vi "GUI AC Source setup.vi"(10 "AC sync source":T2, 11 "AC Source":T2) -> (2 "AC sync source out":T2, 3 "AC Source out":T2)   [LabVIEW 2020]
doc: "GUI to set up the AC source and check connection."
uses:
  General AC source/Type definitions/AC Source.ctl
  General AC source/Type definitions/AC Source type.ctl
  <vilib>/Utility/error.llb/DialogType.ctl
  <vilib>/Utility/error.llb/Error Cluster From Error Code.vi
  <vilib>/ErrorRing/Error Ring.xnode
  external libraries/varilib/varilib.lvlib
panel:
  in  "AC sync Fluke 57XX ignore errors":bool
  in  "Fluke 57XX ignore errors":bool
  out "sync not tested label":string="This device is not yet fully tested!"
  in  "AC sync VISA":refnum<visa-resource-name> caption="VISA"
  in  "AC sync Fluke 57XX wideband output":bool caption="Fluke 57XX wideband output"
  in  "AC sync ref. clock (Hz)":dbl caption="Reference clock (Hz)\nIf set to zero, ref. clock\nis not used." format="%#_6p"
  in  "AC sync type":T1 caption="AC synchronization type"
  in  "Synchronization by AC signal":bool
  in  "Fluke 57XX wideband output":bool
  out "not tested label":string="This device is not yet fully tested!"
  in  "Ref. clock (Hz)":dbl caption="Reference clock (Hz)\nIf set to zero, ref. clock\nis not used." format="%#_6p"
  in  "AC source type":T1
  in  "VISA":refnum<visa-resource-name>
  out "gui_elements":refnum<vi>[](array[refnum])
  out "Status":string
  in  "save_and_quit":bool
  in  "test":bool
  in  "cancel":bool
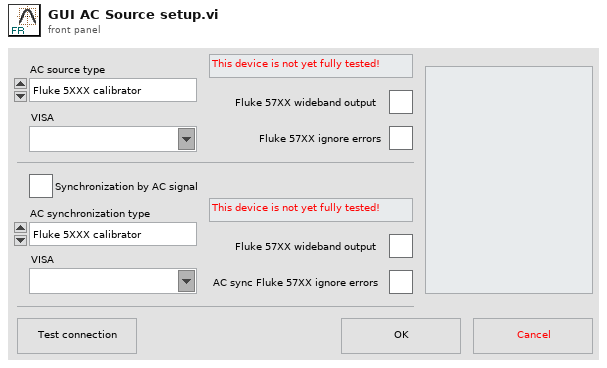
[diagram p1: front panel]
types:
  T1 = typedef "AC Source type.ctl" = enum16{"Fluke 5XXX calibrator", "Tektronix AFG3000 series", "dummy", "Agilent 331xxA to 332xxA", "Agilent 335xxA to 336xxA"}
  T2 = typedef "AC Source.ctl" = cluster{"AC Source type":T1, "VISA":refnum<visa-resource-name>, "Ref. clock (Hz)":dbl, "status ref":refnum<vi>, "Fluke 57XX wideband output":bool, "Fluke 57XX ignore errors":bool, "Synchronization by AC signal":bool}
  T3 = typedef "DialogType.ctl" = u16
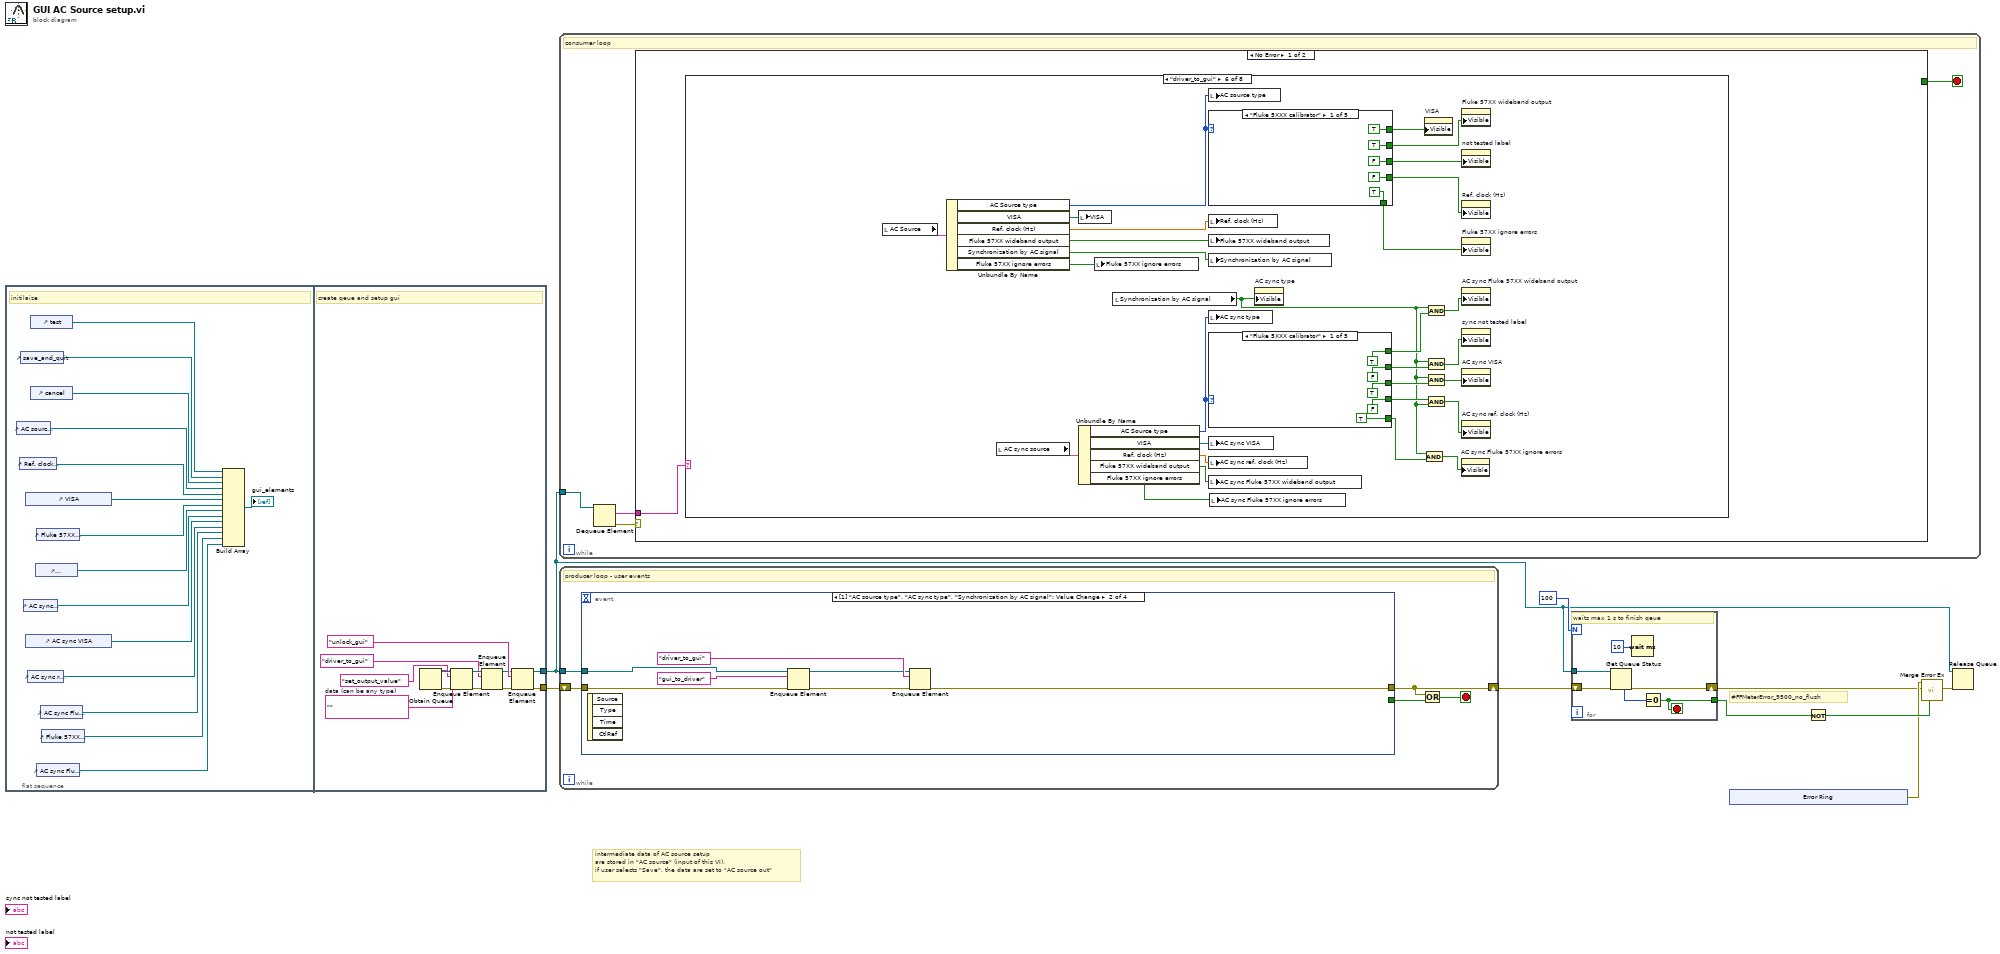
[diagram p0: block diagram]
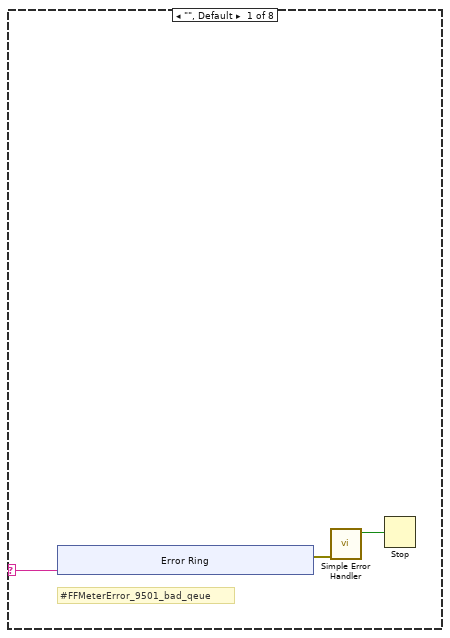
[diagram p2: hidden frame]
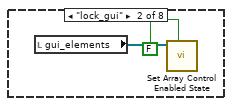
[diagram p3: hidden frame]
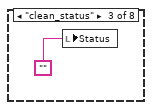
[diagram p4: hidden frame]
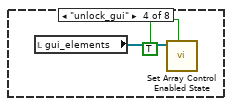
[diagram p5: hidden frame]
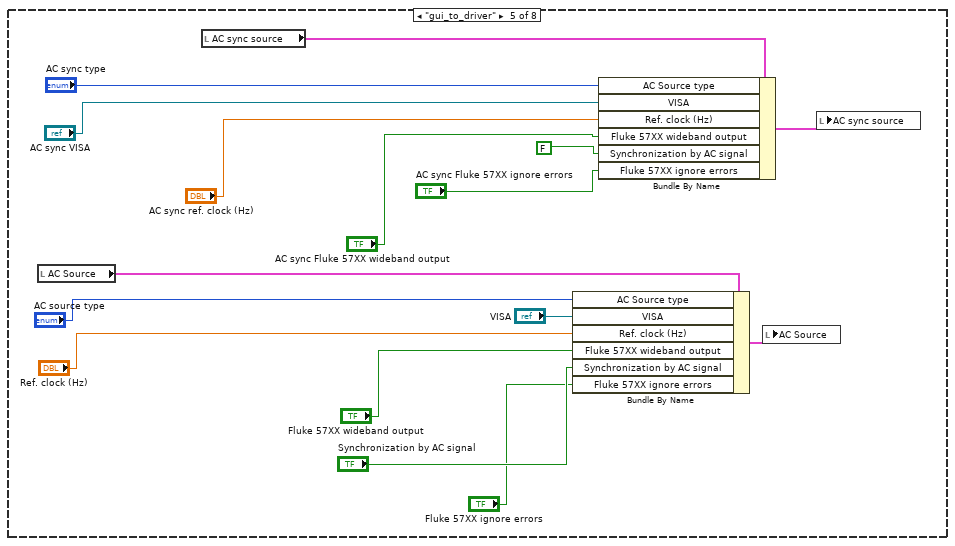
[diagram p6: hidden frame]
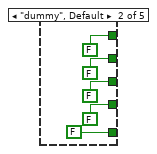
[diagram p7: hidden frame]
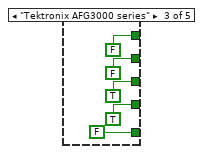
[diagram p8: hidden frame]
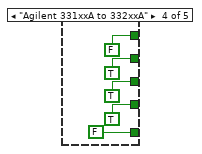
[diagram p9: hidden frame]
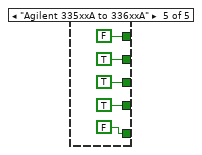
[diagram p10: hidden frame]
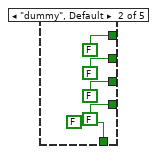
[diagram p11: hidden frame]
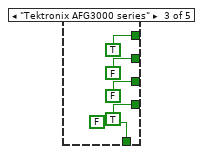
[diagram p12: hidden frame]
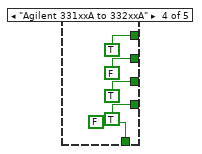
[diagram p13: hidden frame]
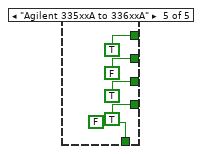
[diagram p14: hidden frame]
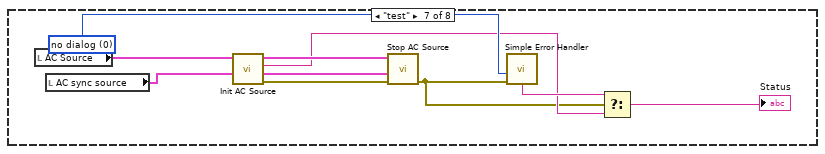
[diagram p15: hidden frame]
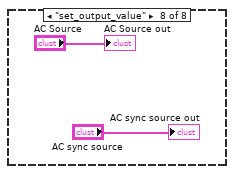
[diagram p16: hidden frame]
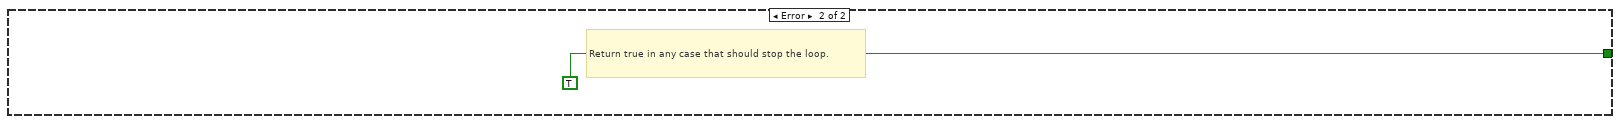
[diagram p17: hidden frame]
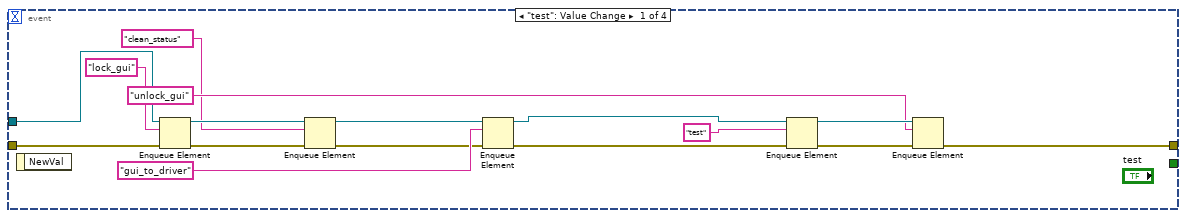
[diagram p18: hidden frame]
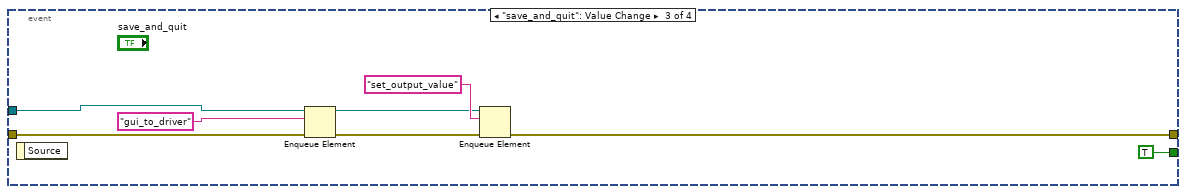
[diagram p19: hidden frame]
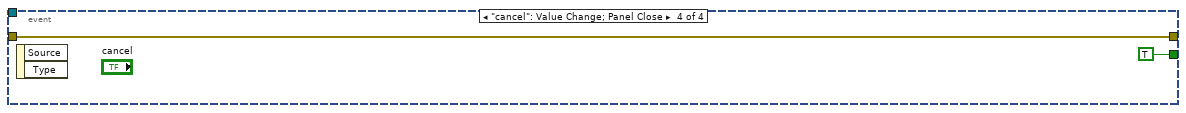
[diagram p20: hidden frame]
diagram:
  # "#FFMeterError_9500_no_flush"
  # "intermediate data of AC source setup\nare stored in \"AC source\" (input of this VI),\nif user selects \"Save\", the data are set to \"AC source out\""
  n1 = flat-sequence {
    tunnel: [w29] -> w2
    tunnel: [w27] -> w1
    frame #0 {
      # "initilaize"
      n2 = control-ref of="AC source type"() -> (w19:refnum<vi>)
      n3 = control-ref of="Ref. clock (Hz)"() -> (w18:refnum<vi>)
      n4 = control-ref of="save_and_quit"() -> (w23:refnum<vi>)
      n5 = control-ref of="AC sync type"() -> (w15:refnum<vi>)
      n6 = control-ref of="VISA"() -> (w20:refnum<vi>)
      n7 = control-ref of="AC sync VISA"() -> (w14:refnum<vi>)
      n8 = control-ref of="AC sync ref. clock (Hz)"() -> (w13:refnum<vi>)
      n9 = control-ref of="test"() -> (w24:refnum<vi>)
      n10 = control-ref of="cancel"() -> (w22:refnum<vi>)
      n11 = control-ref of="Synchronization by AC signal"() -> (w16:refnum<vi>)
      n12 = control-ref of="Fluke 57XX wideband output"() -> (w17:refnum<vi>)
      n13 = control-ref of="AC sync Fluke 57XX ignore errors"() -> (w10:refnum<vi>)
      n14 = control-ref of="AC sync Fluke 57XX wideband output"() -> (w12:refnum<vi>)
      n15 = control-ref of="Fluke 57XX ignore errors"() -> (w11:refnum<vi>)
      n16 = Build Array(w24, w23, w22, w19, w18, w20, w17, w16, w15, w14, w13, w12, w11, w10) -> (→"gui_elements":refnum<vi>[])
    }
    frame #1 {
      w28 = ""  # data (can be any type)
      # "create qeue and setup gui"
      n17 = Obtain Queue(element data type=w28) -> (queue out=w33:refnum<queue>, error out=w35:errorcluster)  [unwired: 4 in, 1 out]
      n18 = Enqueue Element(queue=w33, element="set_output_value", error in (no error)=w35) -> (queue out=w34:refnum<queue>, error out=w36:errorcluster)  [unwired: 1 in, 1 out]
      n19 = Enqueue Element(queue=w34, element="driver_to_gui", error in (no error)=w36) -> (queue out=w25:refnum<queue>, error out=w26:errorcluster)  [unwired: 1 in, 1 out]
      n20 = Enqueue Element(queue=w25, element="unlock_gui", error in (no error)=w26) -> (queue out=w29:refnum<queue>, error out=w27:errorcluster)  [unwired: 1 in, 1 out]
    }
  }
  n21 = while {
    tunnel: w2 -> [w40]
    stop <- w37 stop-if-true
    # "consumer loop"
    n22 = Dequeue Element(queue=w40) -> (element=w38:string, error out=w39:errorcluster)  [unwired: 2 in, 2 out]
    n23 = case shown="No Error" w39 {
      tunnel: w38 -> [w41 _]
      tunnel: [_ TRUE] -> w37
      frame No Error {
        n24 = case shown="\"driver_to_gui\"" w41 {
          selector: w41 -> [w42 _ _ _ _ _ _ _]
          frame "", Default {
            # "#FFMeterError_9501_bad_qeue"
            n25 = xnode "Error Ring"("parameter 0"=w42) -> ("error out"=w44:errorcluster)
            n26 = call <vilib>:"Simple Error Handler.vi"("error in (no error)"=w44) -> ("error?"=w43:bool)  [unwired: 4 in, 4 out]
            n27 = Stop(stop? (T)=w43) -> ()
          }
          frame "lock_gui" {
            n28 = local read "gui_elements"() -> (w53:refnum<vi>[])
            n29 = call "Set Array Control Enabled State.vi"("enabled (T)"=FALSE, "reference array in"=w53) -> ()  [unwired: 8 in, 2 out]
          }
          frame "clean_status" {
            n30 = local write "Status"("") -> ()
          }
          frame "unlock_gui" {
            n31 = local read "gui_elements"() -> (w56:refnum<vi>[])
            n32 = call "Set Array Control Enabled State.vi"("enabled (T)"=TRUE, "reference array in"=w56) -> ()  [unwired: 8 in, 2 out]
          }
          frame "gui_to_driver" {
            n33 = local read "AC Source"() -> (w71:T2)
            n34 = local read "AC sync source"() -> (w65:T2)
            n35 = Bundle By Name(cluster=w71, "AC Source type"="AC source type", "VISA"="VISA", "Ref. clock (Hz)"="Ref. clock (Hz)", "Fluke 57XX wideband output"="Fluke 57XX wideband output", "Synchronization by AC signal"="Synchronization by AC signal", "Fluke 57XX ignore errors"="Fluke 57XX ignore errors") -> (w72:T2)
            n36 = Bundle By Name(cluster=w65, "AC Source type"="AC sync type", "VISA"="AC sync VISA", "Ref. clock (Hz)"="AC sync ref. clock (Hz)", "Fluke 57XX wideband output"="AC sync Fluke 57XX wideband output", "Synchronization by AC signal"=FALSE, "Fluke 57XX ignore errors"="AC sync Fluke 57XX ignore errors") -> (w66:T2)
            n37 = local write "AC Source"(w72) -> ()
            n38 = local write "AC sync source"(w66) -> ()
          }
          frame "driver_to_gui" {
            n39 = local read "AC Source"() -> (w101:T2)
            n40 = Unbundle By Name(w101) -> ("AC Source type"=w100:T1, "VISA"=w97:refnum<visa-resource-name>, "Ref. clock (Hz)"=w99:dbl, "Fluke 57XX wideband output"=w94:bool, "Synchronization by AC signal"=w79:bool, "Fluke 57XX ignore errors"=w78:bool)
            n41 = local read "AC sync source"() -> (w92:T2)
            n42 = local write "VISA"(w97) -> ()
            n43 = Unbundle By Name(w92) -> ("AC Source type"=w88:T1, "VISA"=w91:refnum<visa-resource-name>, "Ref. clock (Hz)"=w90:dbl, "Fluke 57XX wideband output"=w89:bool, "Fluke 57XX ignore errors"=w77:bool)
            n44 = local write "Fluke 57XX ignore errors"(w78) -> ()
            n45 = local read "Synchronization by AC signal"() -> (w75:bool)
            n46 = local write "AC source type"(w100) -> ()
            n47 = case shown="\"Fluke 5XXX calibrator\"" w100 {
              tunnel: [FALSE ("x") FALSE ("x") TRUE ("x") TRUE ("x") TRUE ("x")] -> w96
              tunnel: [TRUE ("x") FALSE ("x") TRUE ("x") TRUE ("x") TRUE ("x")] -> w98
              tunnel: [FALSE ("x") FALSE ("x") FALSE ("x") TRUE ("x") TRUE ("x")] -> w95
              tunnel: [TRUE ("x") FALSE ("x") FALSE ("x") FALSE ("x") FALSE ("x")] -> w93
              tunnel: [TRUE ("x") FALSE ("x") FALSE ("x") FALSE ("x") FALSE ("x")] -> w76
              frame "Fluke 5XXX calibrator" {
              }
              frame "dummy", Default {
              }
              frame "Tektronix AFG3000 series" {
              }
              frame "Agilent 331xxA to 332xxA" {
              }
              frame "Agilent 335xxA to 336xxA" {
              }
            }
            n48 = local write "Ref. clock (Hz)"(w99) -> ()
            n49 = local write "Fluke 57XX wideband output"(w94) -> ()
            n50 = local write "Synchronization by AC signal"(w79) -> ()
            n51 = local write "AC sync type"(w88) -> ()
            n52 = case shown="\"Fluke 5XXX calibrator\"" w88 {
              tunnel: [FALSE ("x") FALSE ("x") TRUE ("x") TRUE ("x") TRUE ("x")] -> w83
              tunnel: [TRUE ("x") FALSE ("x") TRUE ("x") TRUE ("x") TRUE ("x")] -> w87
              tunnel: [FALSE ("x") FALSE ("x") FALSE ("x") TRUE ("x") TRUE ("x")] -> w85
              tunnel: [TRUE ("x") FALSE ("x") FALSE ("x") FALSE ("x") FALSE ("x")] -> w81
              tunnel: [TRUE ("x") FALSE ("x") FALSE ("x") FALSE ("x") FALSE ("x")] -> w74
              frame "Fluke 5XXX calibrator" {
              }
              frame "dummy", Default {
              }
              frame "Tektronix AFG3000 series" {
              }
              frame "Agilent 331xxA to 332xxA" {
              }
              frame "Agilent 335xxA to 336xxA" {
              }
            }
            n53 = local write "AC sync VISA"(w91) -> ()
            n54 = local write "AC sync ref. clock (Hz)"(w90) -> ()
            n55 = local write "AC sync Fluke 57XX wideband output"(w89) -> ()
            n56 = local write "AC sync Fluke 57XX ignore errors"(w77) -> ()
            n57 = property on="AC sync type" class="Enum (strict)"("Visible"=w75) -> ()  [unwired: 2 in, 2 out]
            n58 = And(x=w75, y=w74) -> (x .and. y?=w73:bool)
            n59 = property on="VISA" class="VISAName"("Visible"=w98) -> ()  [unwired: 2 in, 2 out]
            n60 = And(x=w75, y=w81) -> (x .and. y?=w80:bool)
            n61 = And(x=w75, y=w85) -> (x .and. y?=w84:bool)
            n62 = And(x=w75, y=w87) -> (x .and. y?=w86:bool)
            n63 = And(x=w83, y=w75) -> (x .and. y?=w82:bool)
            n64 = property on="AC sync Fluke 57XX ignore errors" class="Bool (strict)"("Visible"=w73) -> ()  [unwired: 2 in, 2 out]
            n65 = property on="Fluke 57XX wideband output" class="Bool (strict)"("Visible"=w93) -> ()  [unwired: 2 in, 2 out]
            n66 = property on="not tested label" class="Str"("Visible"=w95) -> ()  [unwired: 2 in, 2 out]
            n67 = property on="Ref. clock (Hz)" class="DigNum (strict)"("Visible"=w96) -> ()  [unwired: 2 in, 2 out]
            n68 = property on="Fluke 57XX ignore errors" class="Bool (strict)"("Visible"=w76) -> ()  [unwired: 2 in, 2 out]
            n69 = property on="AC sync Fluke 57XX wideband output" class="Bool (strict)"("Visible"=w80) -> ()  [unwired: 2 in, 2 out]
            n70 = property on="sync not tested label" class="Str"("Visible"=w84) -> ()  [unwired: 2 in, 2 out]
            n71 = property on="AC sync VISA" class="VISAName"("Visible"=w86) -> ()  [unwired: 2 in, 2 out]
            n72 = property on="AC sync ref. clock (Hz)" class="DigNum (strict)"("Visible"=w82) -> ()  [unwired: 2 in, 2 out]
          }
          frame "test" {
            w161 = T3 0 items=["no dialog", "OK message", "continue or stop message", "OK message + warnings", "continue/stop + warnings"] ("type of dialog (OK msg:1)")
            n73 = local read "AC Source"() -> (w158:T2)
            n74 = local read "AC sync source"() -> (w153:T2)
            n75 = call "Init AC Source.vi"("AC sync source"=w153, "AC source"=w158) -> ("error out"=w156:errorcluster, "AC sync source out"=w152:T2, "Init status"=w155:string, "AC source out"=w157:T2)  [unwired: 6 in]
            n76 = call "Stop AC Source.vi"("error in (no error)"=w156, "AC sync source"=w152, "AC source"=w157) -> ("error out"=w154:errorcluster)  [unwired: 6 in, 2 out]
            n77 = call <vilib>:"Simple Error Handler.vi"("type of dialog (OK msg:1)"=w161, "error in (no error)"=w154) -> ("message"=w160:string)  [unwired: 3 in, 4 out]
            n78 = Select(t=w160, s=w154, f=w155) -> (s? t:f=→"Status":string)
          }
          frame "set_output_value" {
            "AC Source out" <- "AC Source"
            "AC sync source out" <- "AC sync source"
          }
        }
      }
      frame Error {
        # "Return true in any case that should stop the loop."
      }
    }
  }
  n79 = while {
    shift-right: [w165] -> w5
    shift-left: w1 -> [w168]
    tunnel: w2 -> [w169]
    stop <- w166 stop-if-true
    # "producer loop - user events"
    n80 = event shown="[1] \"AC source type\", \"AC sync type\", \"Synchronization by AC signal\": Value Change" {
      selector: _ -> [_ _ _ _]
      dyn-events: _ -> [_ _ _ _]
      timeout: _ -> [_ _ _ _]
      tunnel: w169 -> [w176 w191 w197 _]
      tunnel: w168 -> [w177 w189 w194 w202]
      tunnel: [w180 w188 w193 w202] -> w165
      tunnel: [_ _ TRUE ("cancel") TRUE ("cancel")] -> w167
      event "test": Value Change {
        n81 = event-data() -> ()  [unwired: 1 in, 1 out]
        n82 = Enqueue Element(queue=w176, element="lock_gui", error in (no error)=w177) -> (queue out=w173:refnum<queue>, error out=w174:errorcluster)  [unwired: 1 in, 1 out]
        n83 = Enqueue Element(queue=w173, element="clean_status", error in (no error)=w174) -> (queue out=w171:refnum<queue>, error out=w172:errorcluster)  [unwired: 1 in, 1 out]
        n84 = Enqueue Element(queue=w171, element="gui_to_driver", error in (no error)=w172) -> (queue out=w183:refnum<queue>, error out=w184:errorcluster)  [unwired: 1 in, 1 out]
        n85 = Enqueue Element(queue=w183, element="test", error in (no error)=w184) -> (queue out=w179:refnum<queue>, error out=w181:errorcluster)  [unwired: 1 in, 1 out]
        n86 = Enqueue Element(queue=w179, element="unlock_gui", error in (no error)=w181) -> (error out=w180:errorcluster)  [unwired: 1 in, 2 out]
      }
      event "Synchronization by AC signal": Value Change {
        n87 = event-data() -> ()  [unwired: 1 in, 4 out]
        n88 = Enqueue Element(queue=w191, element="gui_to_driver", error in (no error)=w189) -> (queue out=w186:refnum<queue>, error out=w187:errorcluster)  [unwired: 1 in, 1 out]
        n89 = Enqueue Element(queue=w186, element="driver_to_gui", error in (no error)=w187) -> (error out=w188:errorcluster)  [unwired: 1 in, 2 out]
      }
      event "save_and_quit": Value Change {
        n90 = event-data() -> ()  [unwired: 1 in, 1 out]
        n91 = Enqueue Element(queue=w197, element="gui_to_driver", error in (no error)=w194) -> (queue out=w196:refnum<queue>, error out=w195:errorcluster)  [unwired: 1 in, 1 out]
        n92 = Enqueue Element(queue=w196, element="set_output_value", error in (no error)=w195) -> (error out=w193:errorcluster)  [unwired: 1 in, 2 out]
      }
      event "cancel": Value Change; Panel Close {
        n93 = event-data() -> ()  [unwired: 1 in, 2 out]
      }
    }
    n94 = Or(x=w165, y=w167) -> (x .or. y?=w166:bool)
  }
  n95 = for {
    N: 100 -> [_]
    tunnel: w2 -> [w208]
    shift-right: [w206] -> w6
    shift-left: w5 -> [w207]
    tunnel: [w203] -> w3
    stop <- w203 stop-if-true
    # "waits max 1 s to finish qeue"
    n96 = Get Queue Status(queue=w208, error in (no error)=w207) -> (error out=w206:errorcluster, # elements in queue=w204:i32)  [unwired: 1 in, 6 out]
    n97 = Wait (ms)(milliseconds to wait=u32 10) -> ()  [unwired: 1 out]
    n98 = Equal To 0?(x=w204) -> (x = 0?=w203:bool)
  }
  n99 = xnode "Error Ring"() -> ("error out"=w7:errorcluster)
  n100 = Not(x=w3) -> (.not. x?=w8:bool)
  n101 = call "Merge Error Ex.vi"("Is error? (False)"=w8, "main error in (no error)"=w6, "second error in"=w7) -> ("error out"=w4:errorcluster)  [unwired: 8 in]
  n102 = Release Queue(queue=w2, error in (no error)=w4) -> ()  [unwired: 1 in, 3 out]
